vi "Smart Parking.vi"() -> ()   [LabVIEW 2013]
panel:
  out "Elapsed Time (s) 2":dbl caption="Elapsed Time (s)"
  in  "Tab Control":enum32{"traffic enforcements", "Client"}(tab)
  out "Sensor 2":bool
  out "Sensor 1":bool
  out "Parking Time":i16
  out "Time left":sgl
  out "Space 1":bool
  out "Incorrectly parked":bool caption="Time has Elapsed"
  out "Time out":bool caption="Time has Elapsed"
  out "Time left to call traffic officer":dbl caption="Elapsed Time (s)"
  out "Time left to call traffic officer":dbl caption="Elapsed Time (s)"
  in  "Coin 1":bool
  out "Space  2":bool
  in  "Coin 2":bool
  out "Time left to call traffic officer":dbl caption="Elapsed Time (s)"
  out "Time left to call traffic officer":dbl caption="Elapsed Time (s)"
  out "Time out":bool caption="Time has Elapsed"
  out "Incorrectly parked":bool caption="Time has Elapsed"
  out "Time left":sgl
  out "Parking Time":i16
  out "Sensor 3":bool
  out "Sensor 4":bool
  out "String":string
  out "Space 1":bool
  out "Time left":sgl
  out "Parking time paid":i16
  out "Incorrectly parked":bool caption="Time has Elapsed"
  out "Perfect parked":bool
  out "Space 2":bool
  out "Perfect parked":bool
  out "Incorrectly parked":bool caption="Time has Elapsed"
  out "Parking time paid":i16
  out "Time left":sgl
  out "String 2":string
  out "Elapsed Time (s)":dbl
  in  "stop":bool
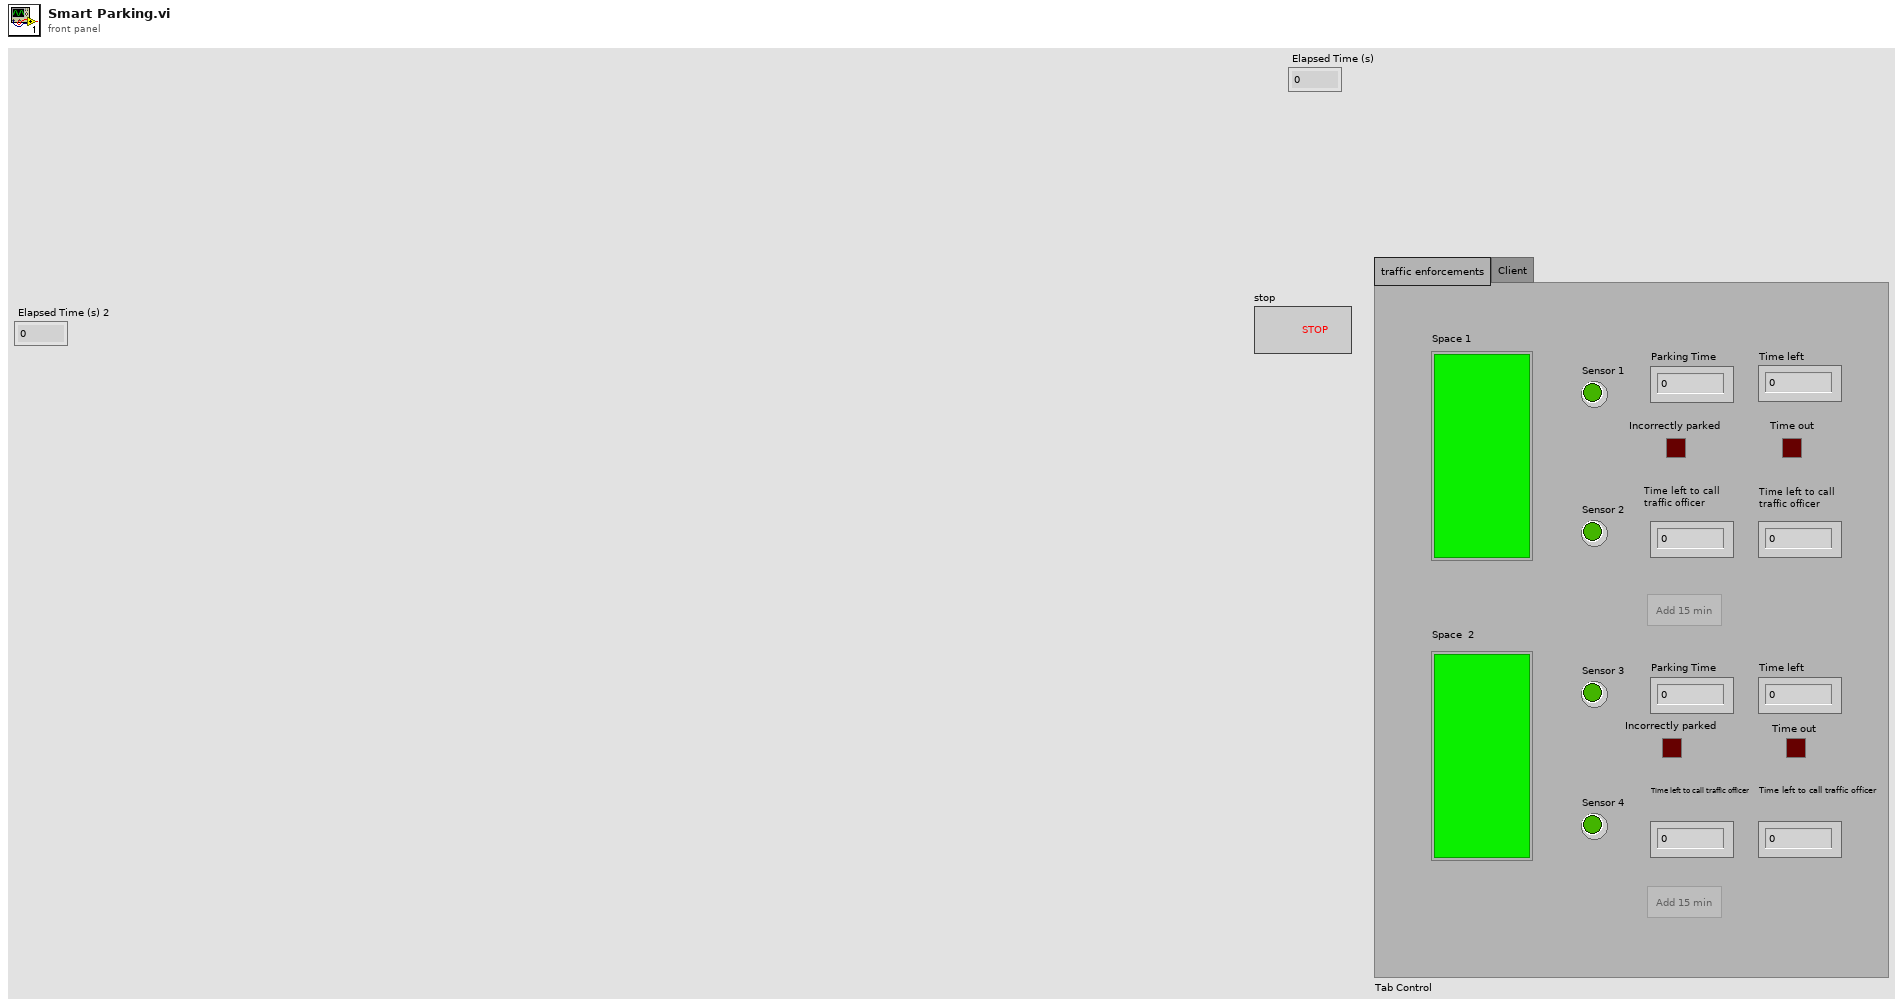
[diagram p1: front panel]
types:
  T1 = enum8{"Enabled", "Disabled", "Disabled and Grayed Out"}
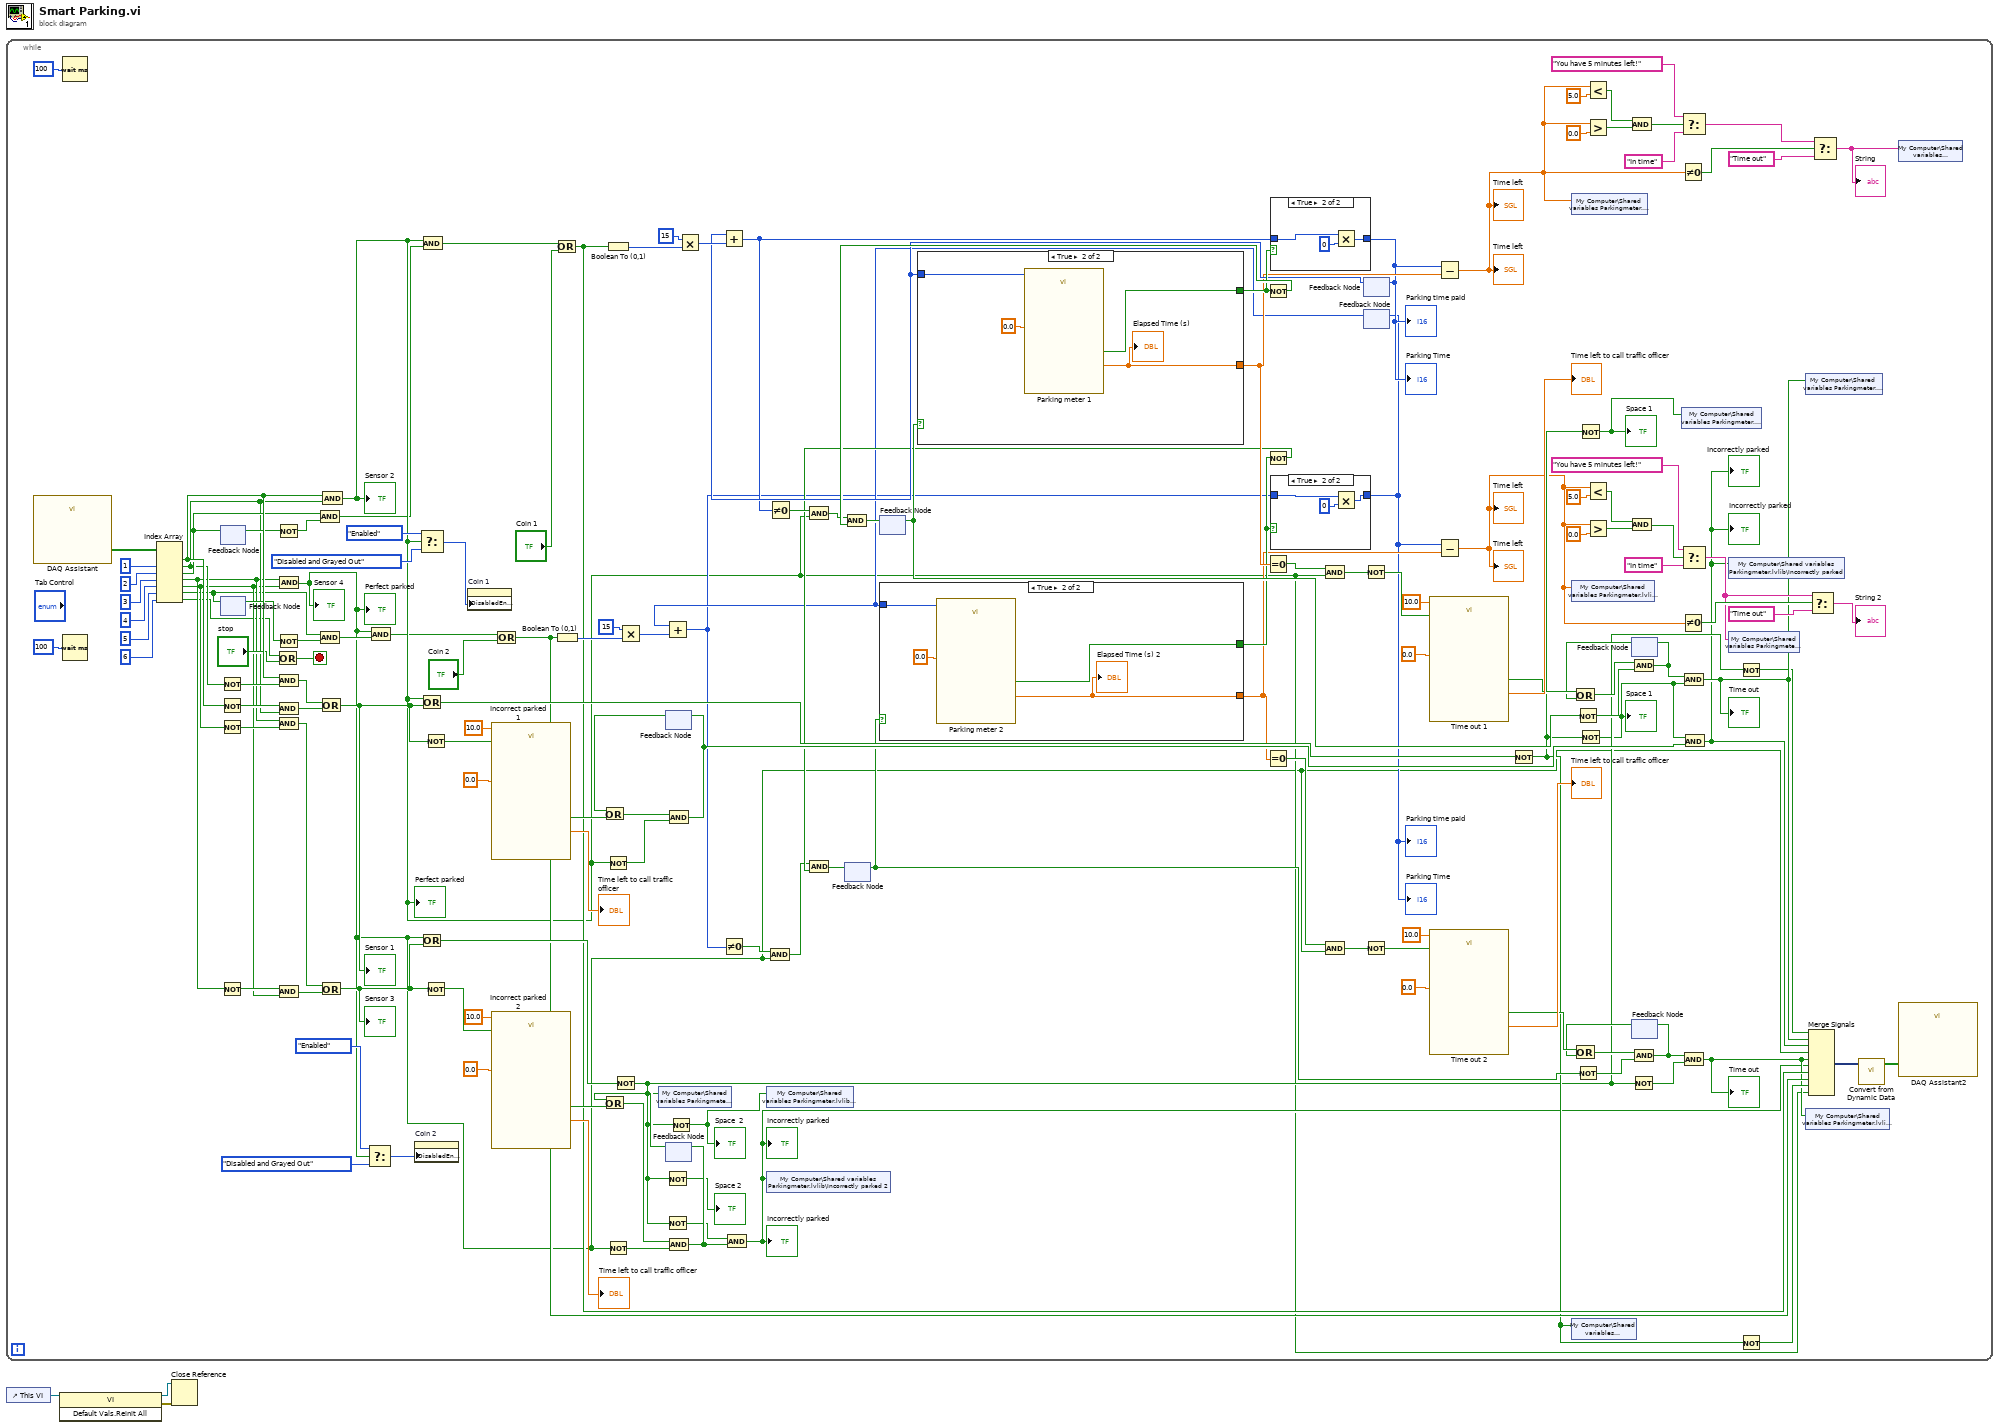
[diagram p0: block diagram]
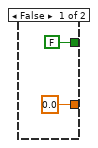
[diagram p3: hidden frame]
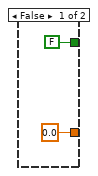
[diagram p5: hidden frame]
diagram:
  n1 = while {
    stop <- w27 stop-if-true
    n2 = call "DAQ Assistant"() -> ("data"=w12:bool[])  [unwired: 17 in, 2 out]
    n3 = Wait (ms)(milliseconds to wait=u32 100) -> ()  [unwired: 1 out]
    n4 = Wait (ms)(milliseconds to wait=u32 100) -> ()  [unwired: 1 out]
    n5 = Index Array(array=w12, index #2=1 ("index"), index #3=2 ("index"), index #4=3 ("index"), index #5=4 ("index"), index #6=5 ("index"), index #7=6 ("index")) -> (element #1=w121:bool, element #2=w16:bool, element #3=w17:bool, element #4=w15:bool, element #5=w14:bool, element #6=w13:bool, element #7=w11:bool)  [unwired: 1 in]
    n6 = Not(x=w16) -> (.not. x?=w159:bool)
    n7 = Not(x=w121) -> (.not. x?=w158:bool)
    n8 = Not(x=w14) -> (.not. x?=w109:bool)
    n9 = Not(x=w15) -> (.not. x?=w108:bool)
    n10 = feedback #1() -> (w117:bool)  [unwired: 1 in]
    n11 = feedback-in #1(w17) -> ()
    n12 = feedback #2() -> (w67:bool)  [unwired: 1 in]
    n13 = feedback-in #2(w13) -> ()
    n14 = Or(x=w11, y="stop") -> (x .or. y?=w27:bool)
    n15 = Not(x=w117) -> (.not. x?=w116:bool)
    n16 = Not(x=w67) -> (.not. x?=w66:bool)
    n17 = And(x=w121, y=w159) -> (x .and. y?=w157:bool)
    n18 = And(x=w158, y=w16) -> (x .and. y?=w156:bool)
    n19 = And(x=w15, y=w109) -> (x .and. y?=w107:bool)
    n20 = And(x=w108, y=w14) -> (x .and. y?=w106:bool)
    n21 = And(x=w15, y=w14) -> (x .and. y?=w4:bool)
    "Sensor 4" <- w4
    "Perfect parked" <- w4
    n22 = And(x=w17, y=w116) -> (x .and. y?=w7:bool)
    n23 = And(x=w13, y=w66) -> (x .and. y?=w5:bool)
    n24 = Or(x=w157, y=w156) -> (x .or. y?=w122:bool)
    "Sensor 1" <- w122
    n25 = Or(x=w107, y=w106) -> (x .or. y?=w72:bool)
    "Sensor 3" <- w72
    n26 = And(x=w121, y=w16) -> (x .and. y?=w8:bool)
    "Sensor 2" <- w8
    "Perfect parked" <- w8
    n27 = Select(t=T1."Enabled" ("Disabled"), s=w4, f=T1."Disabled and Grayed Out" ("Disabled")) -> (s? t:f=w80:T1)
    n28 = And(x=w4, y=w5) -> (x .and. y?=w6:bool)
    n29 = property on="Coin 2" class="Bool"("DisabledEnum"=w80) -> ()  [unwired: 2 in, 2 out]
    n30 = Select(t=T1."Enabled" ("Disabled"), s=w8, f=T1."Disabled and Grayed Out" ("Disabled")) -> (s? t:f=w130:T1)
    n31 = Or(x=w8, y=w122) -> (x .or. y?=w123:bool)
    n32 = Or(x=w4, y=w72) -> (x .or. y?=w73:bool)
    n33 = And(x=w8, y=w7) -> (x .and. y?=w9:bool)
    n34 = Not(x=w122) -> (.not. x?=w141:bool)
    n35 = Not(x=w72) -> (.not. x?=w91:bool)
    n36 = property on="Coin 1" class="Bool"("DisabledEnum"=w130) -> ()  [unwired: 2 in, 2 out]
    n37 = call "Incorrect parked 1"("Time Target (s)"=10.0, "Reset"=w141, "Set Start Time (s)"=0.0) -> ("Elapsed Time (s)"=→"Time left to call traffic officer":dbl, "Time has Elapsed"=w125:bool)  [unwired: 9 in, 6 out]
    n38 = call "Incorrect parked 2"("Time Target (s)"=10.0, "Reset"=w91, "Set Start Time (s)"=0.0) -> ("Elapsed Time (s)"=→"Time left to call traffic officer":dbl, "Time has Elapsed"=w75:bool)  [unwired: 9 in, 6 out]
    n39 = Or(x=w6, y="Coin 2") -> (x .or. y?=w41:bool)
    n40 = Or(x=w9, y="Coin 1") -> (x .or. y?=w57:bool)
    n41 = Boolean To (0,1)(Boolean=w41) -> (0, 1=w103:i16)
    n42 = Boolean To (0,1)(Boolean=w57) -> (0, 1=w153:i16)
    n43 = Not(x=w8) -> (.not. x?=w128:bool)
    n44 = Not(x=w4) -> (.not. x?=w78:bool)
    n45 = Not(x=w73) -> (.not. x?=w33:bool)
    n46 = Multiply(x=i16 15, y=w103) -> (x*y=w104:i16)
    n47 = shared-variable "My Computer\\Shared variables Parkingmeter.lvlib\\Empty 2"(w33) -> ()  [unwired: 1 in, 1 out]
    n48 = Not(x=w33) -> (.not. x?=→"Space 2":bool)
    n49 = Not(x=w33) -> (.not. x?=w63:bool)
    n50 = feedback #3() -> (w127:bool)  [unwired: 1 in]
    n51 = Or(x=w127, y=w125) -> (x .or. y?=w129:bool)
    n52 = And(x=w129, y=w128) -> (x .and. y?=w114:bool)
    n53 = feedback-in #3(w114) -> ()
    n54 = feedback #4() -> (w77:bool)  [unwired: 1 in]
    n55 = Or(x=w77, y=w75) -> (x .or. y?=w79:bool)
    n56 = And(x=w79, y=w78) -> (x .and. y?=w64:bool)
    n57 = feedback-in #4(w64) -> ()
    n58 = Not(x=w33) -> (.not. x?=w35:bool)
    "Space  2" <- w35
    n59 = Multiply(x=i16 15, y=w153) -> (x*y=w154:i16)
    n60 = And(x=w63, y=w64) -> (x .and. y?=w25:bool)
    "Incorrectly parked" <- w25
    "Incorrectly parked" <- w25
    n61 = shared-variable "My Computer\\Shared variables Parkingmeter.lvlib\\Occupied 2"(w35) -> ()  [unwired: 1 in, 1 out]
    n62 = shared-variable "My Computer\\Shared variables Parkingmeter.lvlib\\Incorrectly parked 2"(w25) -> ()  [unwired: 1 in, 1 out]
    n63 = feedback #5() -> (w74:bool)  [unwired: 1 in]
    n64 = feedback #6() -> (w124:bool)  [unwired: 1 in]
    n65 = feedback #7() -> (w146:i16)  [unwired: 1 in]
    n66 = Add(x=w146, y=w154) -> (x+y=w145:i16)
    n67 = Not Equal To 0?(x=w145) -> (x != 0?=w151:bool)
    n68 = And(x=w151, y=w8) -> (x .and. y?=w149:bool)
    n69 = case shown="True" w124 {
      tunnel: [FALSE w178] -> w147
      tunnel: w146 -> [_ w177]
      tunnel: [0.0 ("Elapsed Time (s)") w176] -> w115
      frame False {
      }
      frame True {
        n70 = call "Parking meter 1"("Time Target (s)"=w177, "Set Start Time (s)"=0.0) -> ("Elapsed Time (s)"=w176:dbl, "Time has Elapsed"=w178:bool)  [unwired: 10 in, 6 out]
        "Elapsed Time (s)" <- w176
      }
    }
    n71 = Not(x=w147) -> (.not. x?=w150:bool)
    n72 = And(x=w149, y=w150) -> (x .and. y?=w148:bool)
    n73 = feedback-in #6(w148) -> ()
    n74 = Equal To 0?(x=w115) -> (x = 0?=w138:bool)
    n75 = case shown="True" w147 {
      tunnel: w145 -> [w170 w173]
      tunnel: [w170 w171] -> w113
      frame False {
      }
      frame True {
        n76 = Multiply(x=w173, y=i16 0) -> (x*y=w171:i16)
      }
    }
    "Parking Time" <- w113
    "Parking time paid" <- w113
    n77 = And(x=w138, y=w8) -> (x .and. y?=w136:bool)
    n78 = Not(x=w136) -> (.not. x?=w137:bool)
    n79 = feedback-in #7(w113) -> ()
    n80 = feedback #8() -> (w96:i16)  [unwired: 1 in]
    n81 = Add(x=w96, y=w104) -> (x+y=w95:i16)
    n82 = Not Equal To 0?(x=w95) -> (x != 0?=w101:bool)
    n83 = And(x=w101, y=w4) -> (x .and. y?=w99:bool)
    n84 = case shown="True" w74 {
      tunnel: [FALSE w168] -> w97
      tunnel: w96 -> [_ w167]
      tunnel: [0.0 ("Elapsed Time (s)") w166] -> w65
      frame False {
      }
      frame True {
        n85 = call "Parking meter 2"("Time Target (s)"=w167, "Set Start Time (s)"=0.0) -> ("Elapsed Time (s)"=w166:dbl, "Time has Elapsed"=w168:bool)  [unwired: 10 in, 6 out]
        "Elapsed Time (s) 2" <- w166
      }
    }
    n86 = Not(x=w97) -> (.not. x?=w100:bool)
    n87 = And(x=w99, y=w100) -> (x .and. y?=w98:bool)
    n88 = feedback-in #5(w98) -> ()
    n89 = Equal To 0?(x=w65) -> (x = 0?=w88:bool)
    n90 = case shown="True" w97 {
      tunnel: w95 -> [w160 w163]
      tunnel: [w160 w161] -> w62
      frame False {
      }
      frame True {
        n91 = Multiply(x=w163, y=i16 0) -> (x*y=w161:i16)
      }
    }
    "Parking Time" <- w62
    "Parking time paid" <- w62
    n92 = And(x=w88, y=w4) -> (x .and. y?=w86:bool)
    n93 = Not(x=w86) -> (.not. x?=w87:bool)
    n94 = feedback-in #8(w62) -> ()
    n95 = call "Time out 1"("Time Target (s)"=10.0, "Reset"=w137, "Set Start Time (s)"=0.0) -> ("Elapsed Time (s)"=→"Time left to call traffic officer":dbl, "Time has Elapsed"=w126:bool)  [unwired: 9 in, 6 out]
    n96 = call "Time out 2"("Time Target (s)"=10.0, "Reset"=w87, "Set Start Time (s)"=0.0) -> ("Elapsed Time (s)"=→"Time left to call traffic officer":dbl, "Time has Elapsed"=w76:bool)  [unwired: 9 in, 6 out]
    n97 = Subtract(x=w113, y=w115) -> (x-y=w32:dbl)
    "Time left" <- w32
    "Time left" <- w32
    n98 = Subtract(x=w62, y=w65) -> (x-y=w31:dbl)
    "Time left" <- w31
    "Time left" <- w31
    n99 = Not(x=w123) -> (.not. x?=w34:bool)
    n100 = shared-variable "My Computer\\Shared variables Parkingmeter.lvlib\\Time left"(w32) -> ()  [unwired: 1 in, 1 out]
    n101 = shared-variable "My Computer\\Shared variables Parkingmeter.lvlib\\Time left 2"(w31) -> ()  [unwired: 1 in, 1 out]
    n102 = shared-variable "My Computer\\Shared variables Parkingmeter.lvlib\\Empty"(w34) -> ()  [unwired: 1 in, 1 out]
    n103 = Not(x=w124) -> (.not. x?=w133:bool)
    n104 = Not(x=w74) -> (.not. x?=w83:bool)
    n105 = Not(x=w34) -> (.not. x?=w36:bool)
    "Space 1" <- w36
    n106 = Not(x=w34) -> (.not. x?=w10:bool)
    "Space 1" <- w10
    n107 = Less?(x=w32, y=5.0) -> (x < y?=w53:bool)
    n108 = Greater?(x=w32, y=0.0) -> (0:w56:bool)
    n109 = Less?(x=w31, y=5.0) -> (x < y?=w44:bool)
    n110 = Greater?(x=w31, y=0.0) -> (0:w48:bool)
    n111 = And(x=w53, y=w56) -> (x .and. y?=w55:bool)
    n112 = And(x=w44, y=w48) -> (x .and. y?=w47:bool)
    n113 = Not(x=w33) -> (.not. x?=w71:bool)
    n114 = feedback #9() -> (w120:bool)  [unwired: 1 in]
    n115 = Or(x=w126, y=w120) -> (x .or. y?=w134:bool)
    n116 = And(x=w134, y=w133) -> (x .and. y?=w119:bool)
    n117 = feedback-in #9(w119) -> ()
    n118 = feedback #10() -> (w70:bool)  [unwired: 1 in]
    n119 = Or(x=w76, y=w70) -> (x .or. y?=w84:bool)
    n120 = And(x=w84, y=w83) -> (x .and. y?=w69:bool)
    n121 = feedback-in #10(w69) -> ()
    n122 = Not Equal To 0?(x=w32) -> (x != 0?=w50:bool)
    n123 = Not Equal To 0?(x=w31) -> (x != 0?=w45:bool)
    n124 = Select(t="You have 5 minutes left!", s=w55, f="In time") -> (s? t:f=w52:string)
    n125 = Select(t="You have 5 minutes left!", s=w47, f="In time") -> (s? t:f=w37:string)
    n126 = And(x=w119, y=w10) -> (x .and. y?=w30:bool)
    "Time out" <- w30
    n127 = And(x=w69, y=w71) -> (x .and. y?=w29:bool)
    "Time out" <- w29
    n128 = shared-variable "My Computer\\Shared variables Parkingmeter.lvlib\\Occupied"(w36) -> ()  [unwired: 1 in, 1 out]
    n129 = And(x=w10, y=w114) -> (x .and. y?=w26:bool)
    "Incorrectly parked" <- w26
    "Incorrectly parked" <- w26
    n130 = shared-variable "My Computer\\Shared variables Parkingmeter.lvlib\\Incorrectly parked"(w26) -> ()  [unwired: 1 in, 1 out]
    n131 = shared-variable "My Computer\\Shared variables Parkingmeter.lvlib\\Alarm 2"(w37) -> ()  [unwired: 1 in, 1 out]
    n132 = Not(x=w33) -> (.not. x?=w24:bool)
    n133 = Not(x=w34) -> (.not. x?=w40:bool)
    n134 = shared-variable "My Computer\\Shared variables Parkingmeter.lvlib\\Time out"(w30) -> ()  [unwired: 1 in, 1 out]
    n135 = shared-variable "My Computer\\Shared variables Parkingmeter.lvlib\\Time out 2"(w29) -> ()  [unwired: 1 in, 1 out]
    n136 = Merge Signals(w24, w30, w26, w4, w29, w25, w57, w41, w40, w8) -> (w59:dynamicdata)
    n137 = Select(t=w37, s=w45, f="Time out") -> (s? t:f=→"String 2":string)
    n138 = Select(t=w52, s=w50, f="Time out") -> (s? t:f=w38:string)
    "String" <- w38
    n139 = call "Convert from Dynamic Data"("Dynamic Data Type"=w59) -> ("Array"=w58:bool[])  [unwired: 3 in]
    n140 = shared-variable "My Computer\\Shared variables Parkingmeter.lvlib\\Alarm"(w38) -> ()  [unwired: 1 in, 1 out]
    n141 = call "DAQ Assistant2"("data"=w58) -> ()  [unwired: 17 in, 2 out]
  }
  n142 = control-ref of="This VI"() -> (w3:refnum<vi>)
  n143 = invoke class="VI" method="Default Vals.Reinit All"(reference=w3) -> (reference out=w1:refnum<vi>, error out=w2:errorcluster)  [unwired: 2 in, 1 out]
  n144 = Close Reference(reference=w1, error in (no error)=w2) -> ()  [unwired: 1 out]
